vi "CPP_AoA_Sta_Cal_Equip_Setup.vi"(3 "error in (no error)":errorcluster, 4 "Load VNA State\nFile?":bool=TRUE) -> (2 "VISA resource name out":refnum<visa-resource-name>)   [LabVIEW 2010]
doc: "This VI configures instrument for measurement."
panel:
  out "error out":errorcluster
  in  "Reset? (T: Yes)":bool=TRUE
  in  "ID Query? (T: Yes)":bool=TRUE
  # "Load VNA State? (i.e. Calibration\nFile) is only turned to false when a\nnew network analyzer is being \ncalibrated."
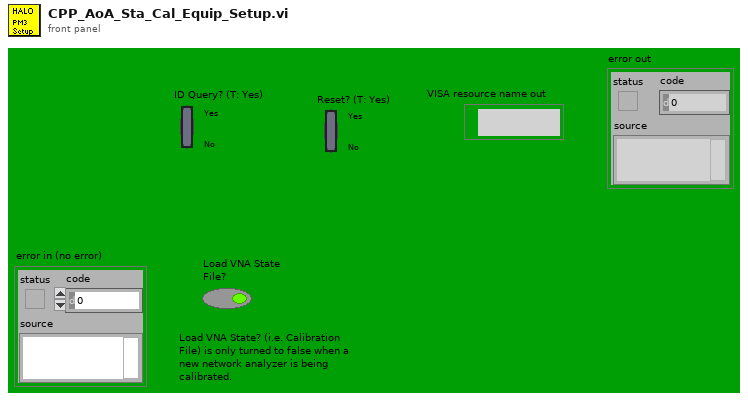
[diagram p1: front panel]
types:
  T1 = enum16{"Single string output", "String Array ouput", "Double Array output", "Decimal Array output"}
  T2 = enum16{"Station parameter", "Product definition", "AOA validation step parameter", "pm2 step parameter", "AOA station cal step parameter", "Station cal Step parameter", "Global variables"}
  T3 = enum16{"single engineering number", "single decimal number", "1D Array input", "string", "2D array input"}
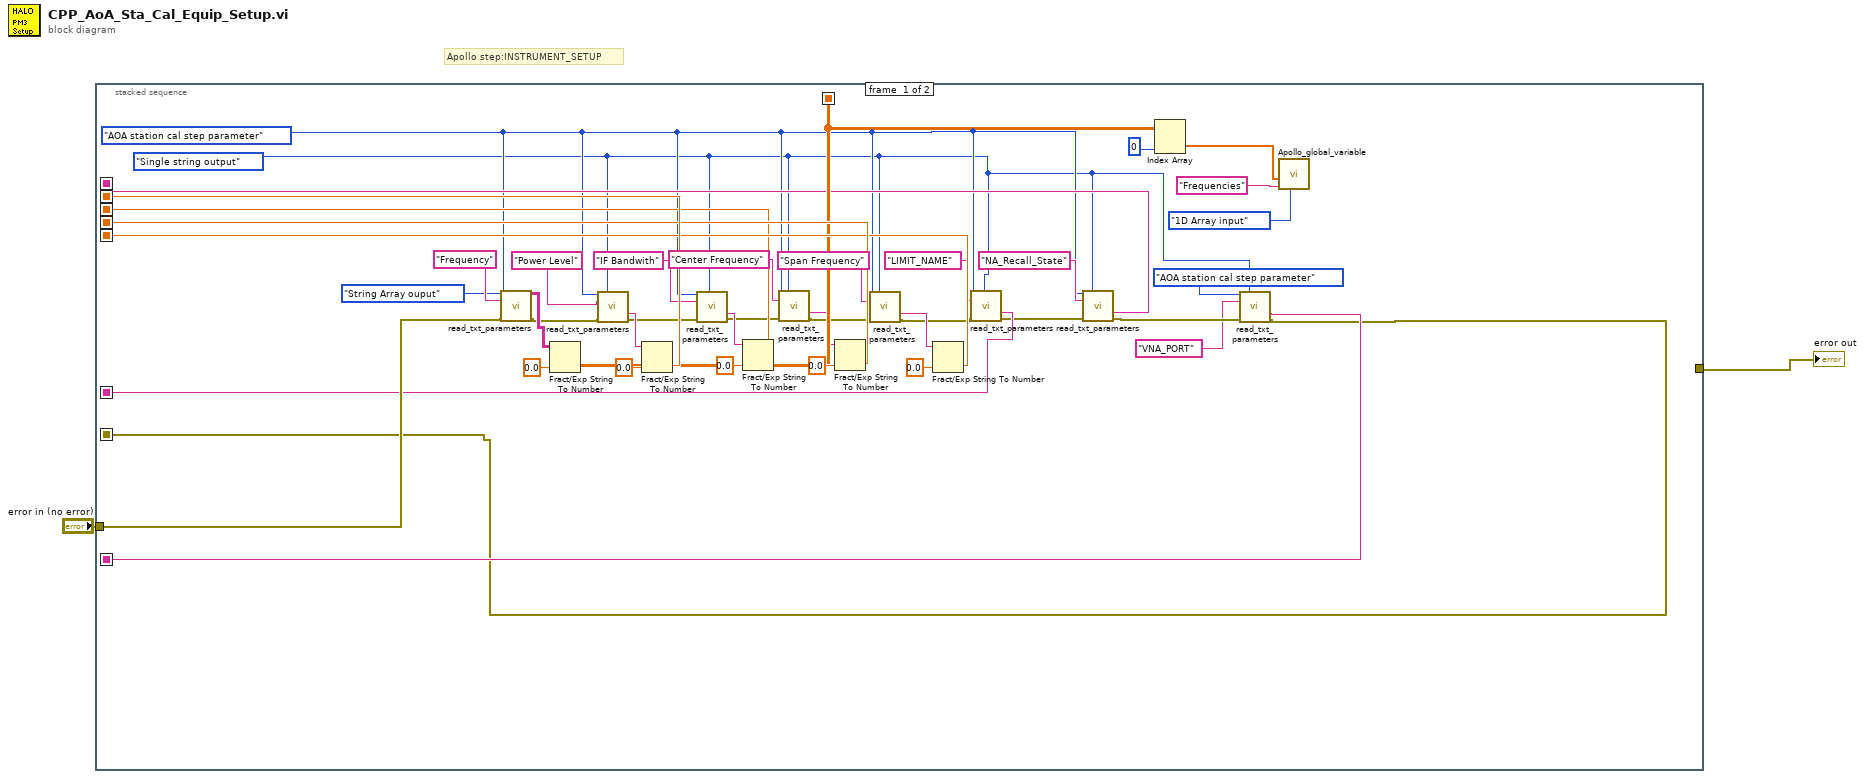
[diagram p0: block diagram]
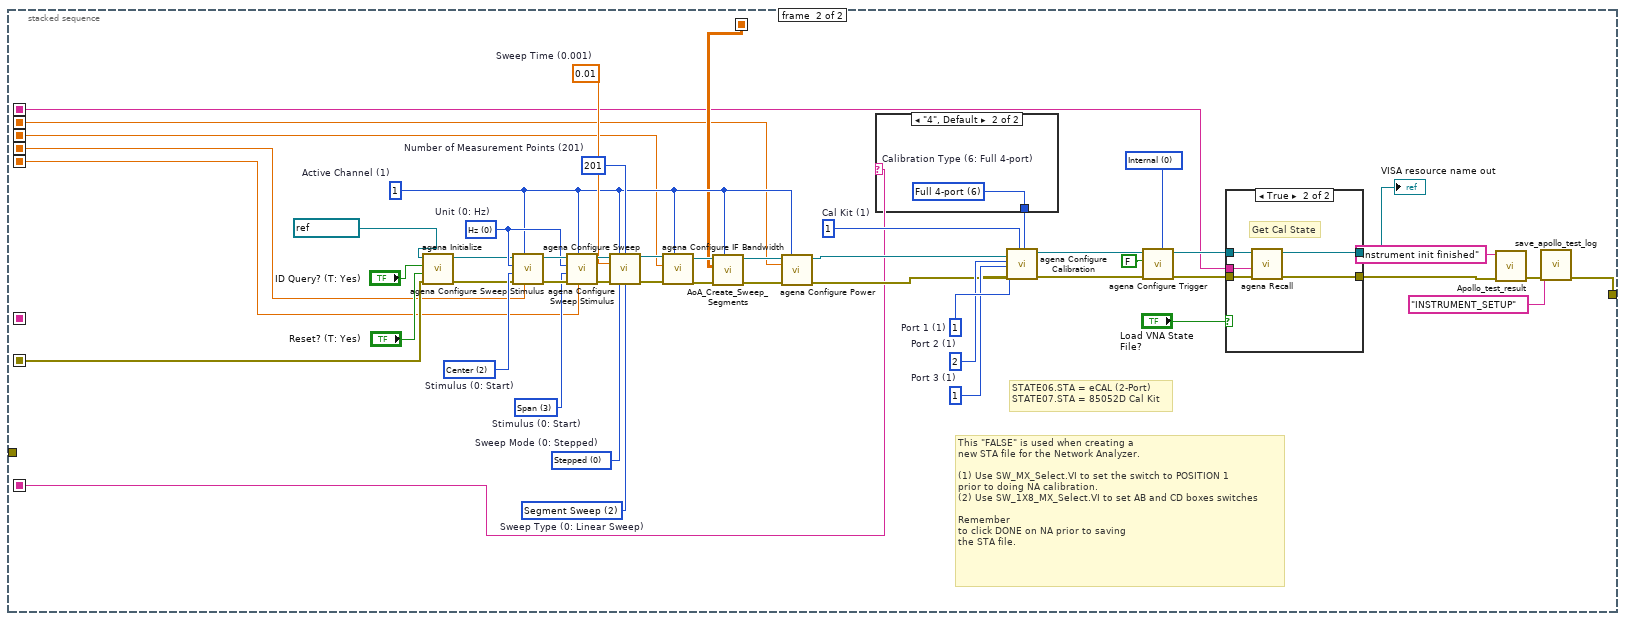
[diagram p2: hidden frame]
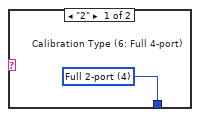
[diagram p3: hidden frame]
diagram:
  # "Apollo step:INSTRUMENT_SETUP"
  n1 = stacked-sequence {
    seq-local: [w10 _] -> [_ w59]
    seq-local: [w36 _] -> [_ w58]
    seq-local: [w45 _] -> [_ w57]
    seq-local: [w37 _] -> [_ w56]
    seq-local: [w39 _] -> [_ w55]
    seq-local: [w38 _] -> [_ w54]
    seq-local: [w20 _] -> [_ _]
    seq-local: [w15 _] -> [_ w53]
    seq-local: [w11 _] -> [_ w52]
    tunnel: "error in (no error)" -> [w33 _]
    tunnel: [_ w49] -> w1
    frame #0 {
      w5 = T1."Single string output" ("Output format")
      w9 = T2."AOA station cal step parameter"
      n2 = call "read_txt_parameters.vi"("Loading mode"=w9, "Output format"=T1."String Array ouput", "file name"="Frequency" ("ParamName"), "error in"=w33) -> ("String Array output"=w35:string[][], "error out"=w31:errorcluster)  [unwired: 7 in, 3 out]
      n3 = Fract/Exp String To Number(string=w35, default (0 dbl)=0.0 ("default (0 DBL)")) -> (number=w36:dbl[][])  [unwired: 2 in, 1 out]
      n4 = call "read_txt_parameters.vi"("Loading mode"=w9, "Output format"=w5, "file name"="Power Level" ("ParamName"), "error in"=w31) -> ("Single string output"=w30:string, "error out"=w29:errorcluster)  [unwired: 7 in, 3 out]
      n5 = Fract/Exp String To Number(string=w30, default (0 dbl)=0.0 ("default (0 DBL)")) -> (number=w45:dbl)  [unwired: 2 in, 1 out]
      n6 = call "read_txt_parameters.vi"("Loading mode"=w9, "Output format"=w5, "file name"="IF Bandwith" ("ParamName"), "error in"=w29) -> ("Single string output"=w27:string, "error out"=w26:errorcluster)  [unwired: 7 in, 3 out]
      n7 = Fract/Exp String To Number(string=w27, default (0 dbl)=0.0 ("default (0 DBL)")) -> (number=w37:dbl)  [unwired: 2 in, 1 out]
      n8 = call "read_txt_parameters.vi"("Loading mode"=w9, "Output format"=w5, "file name"="Center Frequency" ("ParamName"), "error in"=w26) -> ("Single string output"=w25:string, "error out"=w23:errorcluster)  [unwired: 7 in, 3 out]
      n9 = Fract/Exp String To Number(string=w25, default (0 dbl)=0.0 ("default (0 DBL)")) -> (number=w39:dbl)  [unwired: 2 in, 1 out]
      n10 = call "read_txt_parameters.vi"("Loading mode"=w9, "Output format"=w5, "file name"="Span Frequency" ("ParamName"), "error in"=w23) -> ("Single string output"=w21:string, "error out"=w19:errorcluster)  [unwired: 7 in, 3 out]
      n11 = Fract/Exp String To Number(string=w21, default (0 dbl)=0.0 ("default (0 DBL)")) -> (number=w38:dbl)  [unwired: 2 in, 1 out]
      n12 = call "read_txt_parameters.vi"("Loading mode"=w9, "Output format"=w5, "file name"="LIMIT_NAME" ("ParamName"), "error in"=w19) -> ("Single string output"=w20:string, "error out"=w17:errorcluster)  [unwired: 7 in, 3 out]
      n13 = call "read_txt_parameters.vi"("Loading mode"=w9, "Output format"=w5, "file name"="NA_Recall_State" ("ParamName"), "error in"=w17) -> ("Single string output"=w15:string, "error out"=w13:errorcluster)  [unwired: 7 in, 3 out]
      n14 = Index Array(array=w36, index (col)=0 ("disabled index (col)")) -> (element=w8:dbl[])  [unwired: 1 in]
      n15 = call "read_txt_parameters.vi"("Loading mode"=T2."AOA station cal step parameter", "Output format"=w5, "file name"="VNA_PORT", "error in"=w13) -> ("Single string output"=w11:string, "error out"=w10:errorcluster)  [unwired: 7 in, 3 out]
      n16 = call "Apollo_global_variable.vi"("Global variable types"=T3."1D Array input", "variable name"="Frequencies", "1D Array input"=w8) -> ()  [unwired: 9 in]
    }
    frame #1 {
      w71 = 0.01  # Sweep Time (0.001)
      w72 = u16 0 items=["Internal", "External", "Manual", "BUS"] ("Trigger Source (0: Internal)")
      w78 = 1  # Cal Kit (1)
      w79 = 2  # Port 2 (1)
      w80 = 1  # Port 3 (1)
      w81 = 1  # Port 1 (1)
      w89 = u16 2 items=["Linear Sweep", "Logaritmic Sweep", "Segment Sweep", "Power Sweep"]  # Sweep Type (0: Linear Sweep)
      w90 = 201  # Number of Measurement Points (201)
      w91 = u16 0 items=["Stepped", "Swept", "Fast Stepped Mode", "Fast Swept Mode"]  # Sweep Mode (0: Stepped)
      w93 = u16 3 items=["Start", "Stop", "Center", "Span"]  # Stimulus (0: Start)
      w92 = u16 0 items=["Hz", "kHz", "MHz", "GHz", "dBm", "s"]  # Unit (0: Hz)
      w96 = u16 2 items=["Start", "Stop", "Center", "Span"]  # Stimulus (0: Start)
      w66 = 1  # Active Channel (1)
      # "This \"FALSE\" is used when creating a \nnew STA file for the Network Analyzer.\n\n(1) Use SW_MX_Select.VI to set the switch to POSITION 1\nprior to doing NA calibration.  \n(2) Use SW_1X8_MX_Select.VI to set AB and CD boxes switches\n\nRemember \nto click DONE on NA prior to saving\nthe STA file."
      # "STATE06.STA = eCAL (2-Port)\nSTATE07.STA = 85052D Cal Kit"
      n17 = call "agena Initialize.vi"("error in (no error)"=w59, "Reset? (T: Yes)"="Reset? (T: Yes)", "ID Query? (T: Yes)"="ID Query? (T: Yes)", "VISA resource name"=refnum<visa-resource-name> "E5071C" ("Vector Network Analyzer \nVISA resource name")) -> ("error out"=w83:errorcluster, "VISA resource name out"=w84:refnum<visa-resource-name>)  [unwired: 6 in]
      n18 = call "agena Configure Sweep Stimulus.vi"("Parameter (0.0)"=w55, "Channel (1)"=w66, "error in (no error)"=w83, "Stimulus (0: Start)"=w96, "Unit (0: Hz)"=w92, "VISA resource name"=w84) -> ("error out"=w95:errorcluster, "VISA resource name out"=w94:refnum<visa-resource-name>)  [unwired: 4 in]
      n19 = call "agena Configure Sweep Stimulus.vi"("Parameter (0.0)"=w54, "Channel (1)"=w66, "error in (no error)"=w95, "Stimulus (0: Start)"=w93, "Unit (0: Hz)"=w92, "VISA resource name"=w94) -> ("error out"=w88:errorcluster, "VISA resource name out"=w87:refnum<visa-resource-name>)  [unwired: 4 in]
      n20 = call "agena Configure Sweep.vi"("VISA resource name"=w87, "Channel (1)"=w66, "Number of Measurement Points (201)"=w90, "Sweep Time (0.001)"=w71, "error in (no error)"=w88, "Sweep Mode (0: Stepped)"=w91, "Sweep Type (0: Linear Sweep)"=w89) -> ("VISA resource name out"=w86:refnum<visa-resource-name>, "error out"=w85:errorcluster)  [unwired: 7 in]
      n21 = call "agena Configure IF Bandwidth.vi"("Channel (1)"=w66, "error in (no error)"=w85, "IF Bandwidth (100000.0)"=w56, "VISA resource name"=w86) -> ("error out"=w69:errorcluster, "VISA resource name out"=w70:refnum<visa-resource-name>)  [unwired: 6 in]
      n22 = call "AoA_Create_Sweep_Segments.vi"("Channel (1)"=w66, "error in"=w69, "Frequency"=w58, "VISA resource name"=w70) -> ("error out"=w67:errorcluster, "VISA resource name out"=w68:refnum<visa-resource-name>)  [unwired: 4 in]
      n23 = call "agena Configure Power.vi"("VISA resource name"=w68, "Channel (1)"=w66, "Power Level (0.0)"=w57, "error in (no error)"=w67) -> ("VISA resource name out"=w65:refnum<visa-resource-name>, "error out"=w64:errorcluster)  [unwired: 10 in]
      n24 = case shown="\"4\", Default" w52 {
        tunnel: [w97 w98] -> w82
        frame "2" {
          w97 = u16 4 items=["Open", "Short", "Through", "1-port", "Full 2-port", "Full 3-port", "Full 4-port"]  # Calibration Type (6: Full 4-port)
        }
        frame "4", Default {
          w98 = u16 6 items=["Open", "Short", "Through", "1-port", "Full 2-port", "Full 3-port", "Full 4-port"]  # Calibration Type (6: Full 4-port)
        }
      }
      n25 = call "agena Configure Calibration.vi"("VISA resource name"=w65, "Port 1 (1)"=w81, "Port 2 (1)"=w79, "Port 3 (1)"=w80, "error in (no error)"=w64, "Cal Kit (1)"=w78, "Calibration Type (6: Full 4-port)"=w82) -> ("VISA resource name out"=w74:refnum<visa-resource-name>, "error out"=w75:errorcluster)  [unwired: 11 in]
      n26 = call "agena Configure Trigger.vi"("Trigger Source (0: Internal)"=w72, "error in (no error)"=w75, "Continuous Sweep (T: Enable)"=FALSE, "VISA resource name"=w74) -> ("error out"=w62:errorcluster, "VISA resource name out"=w63:refnum<visa-resource-name>)  [unwired: 6 in]
      n27 = case shown="True" "Load VNA State\nFile?" {
        tunnel: w63 -> [w100 w105]
        tunnel: w62 -> [w99 w104]
        tunnel: [w100 w103] -> w61
        tunnel: [w99 w102] -> w48
        tunnel: w53 -> [_ w101]
        frame False {
        }
        frame True {
          # "Get Cal State"
          n28 = call "agena Recall.vi"("error in (no error)"=w104, "File Name ()"=w101, "VISA resource name"=w105) -> ("error out"=w102:errorcluster, "VISA resource name out"=w103:refnum<visa-resource-name>)  [unwired: 7 in]
        }
      }
      "VISA resource name out" <- w61
      n29 = call "Apollo_test_result.vi"("Test Message"="Instrument init finished", "error in"=w48) -> ("error out"=w50:errorcluster)  [unwired: 3 in]
      n30 = call "save_apollo_test_log.vi"("error in (no error)"=w50, "Test name"="INSTRUMENT_SETUP") -> ("error out"=w49:errorcluster)  [unwired: 9 in]
    }
  }
  "error out" <- w1
